vi "Intake_Execute.vi"() -> ()   [LabVIEW 2019]
uses:
  <vilib>/Rock Robotics/WPI/ThirdParty/REV Robotics/SPARK MAX/Typedef/Spark MAX Control Type.ctl
  <vilib>/Rock Robotics/WPI/Solenoid/WPI_SolenoidValue.ctl
  Intake_Cluster.ctl
  Intake_States.ctl
  Globals/Intake_Globals.vi
  Globals/Solenoid Globals.vi
  <vilib>/Rock Robotics/WPI/Solenoid/WPI_SolenoidSetEnum.vi
panel:
  in  "Intake_Speed":dbl=0.45
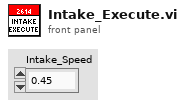
[diagram p1: front panel]
types:
  T1 = typedef "WPI_MotorControlDeviceRef.ctl" = cluster{"DeviceStatus":errorcluster, "Type":T2, "PWM":cluster{"PWM Channel":T3, "DeadBand":T4}, "CAN":cluster{"Device Number":u8, "SetOutput VI Ref":variant, "GetOutput VI Ref":variant, "Enable VI Ref":variant, "Disable VI Ref":variant, "Data":variant}, "Invert":bool, "DIO PWM":cluster{"PWM \"Enable\" Channel":T3, "DIOChannel":T5, "PWM Rate":dbl}}
  T2 = typedef "WPI_MotorControlType.ctl" = enum16{"PWM", "CAN", "DIO PWM"}
  T3 = typedef "FPGA_DIOPWMChannel.ctl" = enum8{"PWM 0", "PWM 1", "PWM 2", "PWM 3", "PWM 4", "PWM 5", "PWM 6", "PWM 7", "PWM 8", "PWM 9", "PWM MXP 0", "PWM MXP 1", "PWM MXP 2", "PWM MXP 3", "PWM MXP 4", "PWM MXP 5", "PWM MXP 6", "PWM MXP 7", "PWM MXP 8", "PWM MXP 9", "Invalid"}
  T4 = typedef "WPI_PWMDeadband.ctl" = cluster{"Name":string, "maxPositivePwm":i32, "minPositivePwm":i32, "centerPwm":i32, "maxNegativePwm":i32, "minNegativePwm":i32, "angularRange":u16}
  T5 = typedef "FPGA_DIOChannel.ctl" = enum8{"DIO 0", "DIO 1", "DIO 2", "DIO 3", "DIO 4", "DIO 5", "DIO 6", "DIO 7", "DIO 8", "DIO 9", "DIO MXP 0", "DIO MXP 1", "DIO MXP 2", "DIO MXP 3", "DIO MXP 4", "DIO MXP 5", "DIO MXP 6", "DIO MXP 7", "DIO MXP 8", "DIO MXP 9", "DIO MXP 10", "DIO MXP 11", "DIO MXP 12", "DIO MXP 13", "DIO MXP 14", "DIO MXP 15", "SPI Port CS1", "SPI Port CS2", "SPI Port CS3", "SPI Port MISO", "SPI Port MOSI", "Invalid"}
  T6 = typedef "WPI_SolenoidDevRef.ctl" = cluster{"DevStatus":errorcluster, "Pneumatics Control Module":u8, "Forward Solenoid Channel":T7, "Reverse Solenoid Channel":T7}
  T7 = typedef "WPI_SolenoidChannel.ctl" = enum8{"Solenoid 0", "Solenoid 1", "Solenoid 2", "Solenoid 3", "Solenoid 4", "Solenoid 5", "Solenoid 6", "Solenoid 7", "Invalid"}
  T8 = typedef "WPI_SolenoidValue.ctl" = enum16{"Off", "On", "Forward", "Reverse"}
  T9 = typedef "Intake_Cluster.ctl" = cluster{"Control_State":T10, "Intake_On":bool, "Intake_Extended":bool, "Intake_Throttle":dbl, "Auto_Notifier":refnum<notifier>, "Parameter_1":dbl, "Parameter_2":dbl, "Step":dbl, "Outtake":bool}
  T10 = typedef "Intake_States.ctl" = enum16{"Manual_Control", "Compliant_Intake", "Command_RunIntake"}
  T11 = typedef "Spark MAX Control Type.ctl" = enum16{"Percent VBus", "Voltage", "Velocity", "Position", "Smart Motion", "Current", "Smart Velocity"}
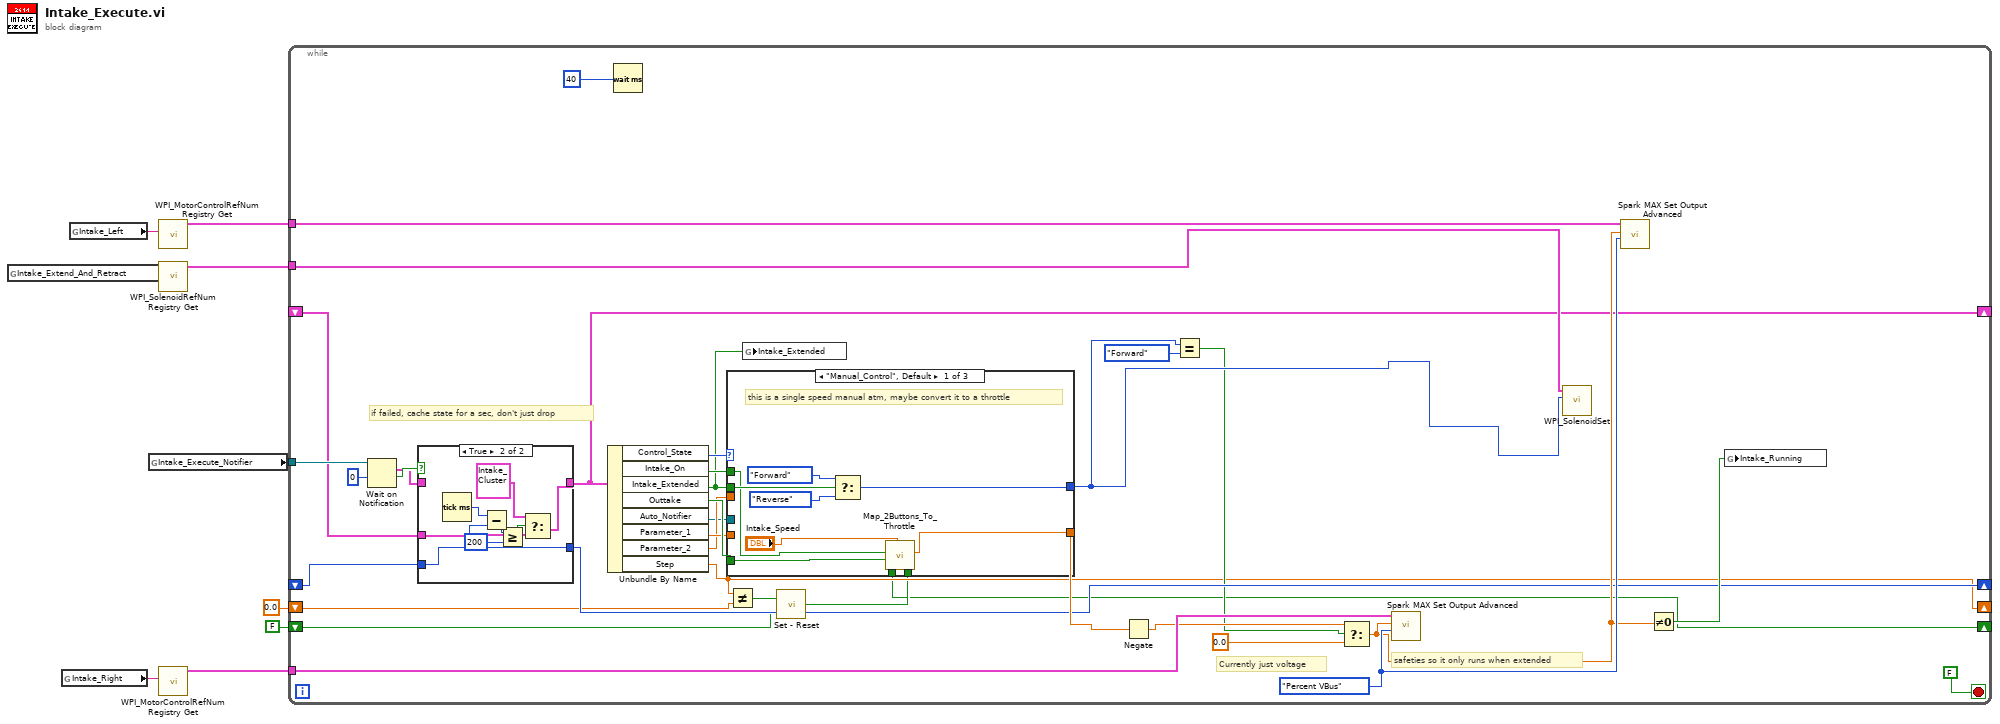
[diagram p0: block diagram]
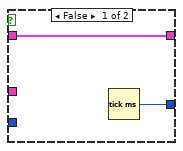
[diagram p2: hidden frame]
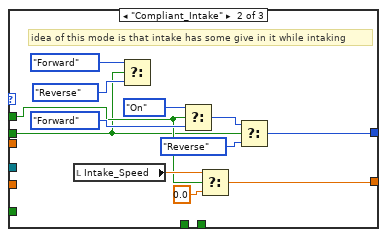
[diagram p3: hidden frame]
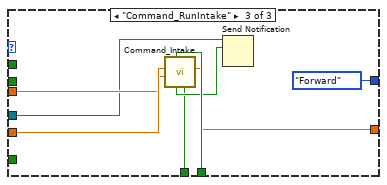
[diagram p4: hidden frame]
diagram:
  n1 = global read "Solenoid Globals.vi" "Intake_Extend_And_Retract"() -> (w4:string)
  n2 = global read "Intake_Globals.vi" "Intake_Right"() -> (w8:string)
  n3 = global read "Intake_Globals.vi" "Intake_Left"() -> (w7:string)
  n4 = global read "Intake_Globals.vi" "Intake_Execute_Notifier"() -> (w9:refnum<notifier>)
  n5 = call <vilib>:"WPI_MotorControlRefNum Registry Get.vi"("refnum name"=w7) -> ("MotorControlDevRef"=w6:T1)  [unwired: 9 in, 1 out]
  n6 = call <vilib>:"WPI_SolenoidRefNum Registry Get.vi"("refnum name"=w4) -> ("SolenoidDevRef"=w3:T6)  [unwired: 9 in, 1 out]
  n7 = call <vilib>:"WPI_MotorControlRefNum Registry Get.vi"("refnum name"=w8) -> ("MotorControlDevRef"=w5:T1)  [unwired: 9 in, 1 out]
  n8 = while {
    tunnel: w9 -> [w43]
    tunnel: w6 -> [w39]
    tunnel: w5 -> [w38]
    tunnel: w3 -> [w36]
    shift-right: [w24] -> _
    shift-left: _ -> [w23]
    shift-right: [w22] -> _
    shift-left: _ -> [w21]
    shift-right: [w16] -> _
    shift-left: 0.0 ("Step") -> [w15]
    shift-right: [w11] -> _
    shift-left: FALSE ("Reint") -> [w13]
    stop <- FALSE stop-if-true
    w37 = Spark_MAX_Control_Type."Percent VBus" ("Control Mode")
    # "if failed, cache state for a sec, don't just drop"
    # "Currently just voltage"
    # "safeties so it only runs when extended"
    n9 = Wait on Notification(notifier=w43, timeout in ms (-1)=0) -> (notification=w25:T9, timed out?=w27:bool)  [unwired: 2 in, 2 out]
    n10 = case shown="True" w27 {
      tunnel: w25 -> [w46 _]
      tunnel: [w46 w54] -> w24
      tunnel: w23 -> [_ w53]
      tunnel: [w45 w51] -> w22
      tunnel: w21 -> [_ w51]
      frame False {
        n11 = Tick Count (ms)() -> (millisecond timer value=w45:u32)
      }
      frame True {
        n12 = Tick Count (ms)() -> (millisecond timer value=w52:u32)
        n13 = Subtract(x=w52, y=w51) -> (x-y=w49:u32)
        n14 = Greater Or Equal?(x=w49, y=u32 200) -> (x >= y?=w50:bool)
        n15 = Select(t=T9 {"Control_State"=enum."Manual_Control", "Intake_On"=FALSE, "Intake_Extended"=FALSE, "Intake_Throttle"=0.0, "Auto_Notifier"=refnum, "Parameter_1"=0.0, "Parameter_2"=0.0, "Step"=0.0, "Outtake"=FALSE}, s=w50, f=w53) -> (s? t:f=w54:T9)
      }
    }
    n16 = Unbundle By Name(w24) -> ("Control_State"=w42:T10, "Intake_On"=w41:bool, "Intake_Extended"=w10:bool, "Outtake"=w33:bool, "Auto_Notifier"=w17:refnum<notifier>, "Parameter_1"=w19:dbl, "Parameter_2"=w18:dbl, "Step"=w16:dbl)
    n17 = Wait (ms)(milliseconds to wait=u32 40) -> ()  [unwired: 1 out]
    n18 = Not Equal?(x=w16, y=w15) -> (x != y?=w14:bool)
    n19 = global write "Intake_Globals.vi" "Intake_Extended"(w10) -> ()
    n20 = call "Set - Reset.vi"("Reset"=w13, "Set"=w14) -> ("Output"=w12:bool)
    n21 = case shown="\"Manual_Control\", Default" w42 {
      tunnel: w10 -> [w59 w64 _]
      tunnel: [w60 w71 WPI_SolenoidValue."Forward" ("Value")] -> w32
      tunnel: w41 -> [w58 w67 _]
      tunnel: [w55 w63 w76] -> w31
      tunnel: w33 -> [w57 _ _]
      tunnel: w19 -> [_ _ w82]
      tunnel: w18 -> [_ _ w81]
      tunnel: w17 -> [_ _ w80]
      tunnel: w12 -> [_ _ w79]
      tunnel: [_ _ w77] -> w11
      frame "Manual_Control", Default {
        # "this is a single speed manual atm, maybe convert it to a throttle"
        n22 = Select(t=WPI_SolenoidValue."Forward" ("Value"), s=w59, f=WPI_SolenoidValue."Reverse" ("Value")) -> (s? t:f=w60:T8)
        n23 = call "Map_2Buttons_To_Throttle.vi"("Power"="Intake_Speed", "Down"=w57, "Up"=w58) -> ("Throttle"=w55:dbl)  [unwired: 8 in]
      }
      frame "Compliant_Intake" {
        # "idea of this mode is that intake has some give in it while intaking"
        n24 = local read "Intake_Speed"() -> (w72:dbl)
        n25 = Select(t=WPI_SolenoidValue."Forward" ("Value"), s=w64, f=WPI_SolenoidValue."Reverse" ("Value")) -> ()  [unwired: 1 out]
        n26 = Select(t=WPI_SolenoidValue."On" ("Value"), s=w67, f=WPI_SolenoidValue."Forward" ("Value")) -> (s? t:f=w70:T8)
        n27 = Select(t=w72, s=w67, f=0.0) -> (s? t:f=w63:dbl)
        n28 = Select(t=w70, s=w64, f=WPI_SolenoidValue."Reverse" ("Value")) -> (s? t:f=w71:T8)
      }
      frame "Command_RunIntake" {
        n29 = call "Command_Intake.vi"("Startup"=w79, "Timeout"=w81, "Speed"=w82) -> ("Intake_Output"=w76:dbl, "Reint"=w77:bool, "Completed"=w78:bool)  [unwired: 6 in]
        n30 = Send Notification(notification=w78, notifier=w80) -> ()  [unwired: 1 in, 2 out]
      }
    }
    n31 = Negate(x=w31) -> (-x=w30:dbl)
    n32 = Equal?(x=w32, y=WPI_SolenoidValue."Forward") -> (x = y?=w20:bool)
    n33 = Select(t=w30, s=w20, f=0.0) -> (s? t:f=w29:dbl)
    n34 = call <vilib>:"Spark MAX Set Output Advanced.vi"("Control Mode"=w37, "Setpoint"=w29, "MotorControlDevRef"=w38) -> ()  [unwired: 7 in, 2 out]
    n35 = call-poly <vilib>:"WPI_SolenoidSet.vi"("Value"=w32, "SolenoidDevRef"=w36) -> ()  [unwired: 8 in, 2 out]
    n36 = call <vilib>:"Spark MAX Set Output Advanced.vi"("Control Mode"=w37, "Setpoint"=w29, "MotorControlDevRef"=w39) -> ()  [unwired: 7 in, 2 out]
    n37 = Not Equal To 0?(x=w29) -> (x != 0?=w28:bool)
    n38 = global write "Intake_Globals.vi" "Intake_Running"(w28) -> ()
  }
